vi "trial 1.vi"() -> ()   [LabVIEW 2013]
uses:
  <vilib>/vision/NI_Vision_Development_Module.lvlib
panel:
  in  "Contours 2":T1(array[cluster])
  in  "Global Rectangle 2":i32[](array[numeric])
  out "Contours":T1(array[cluster])
  out "Global Rectangle":i32[](array[numeric])
  out "Image 3":T2(plugin-control)
  in  "AVI File Path":path
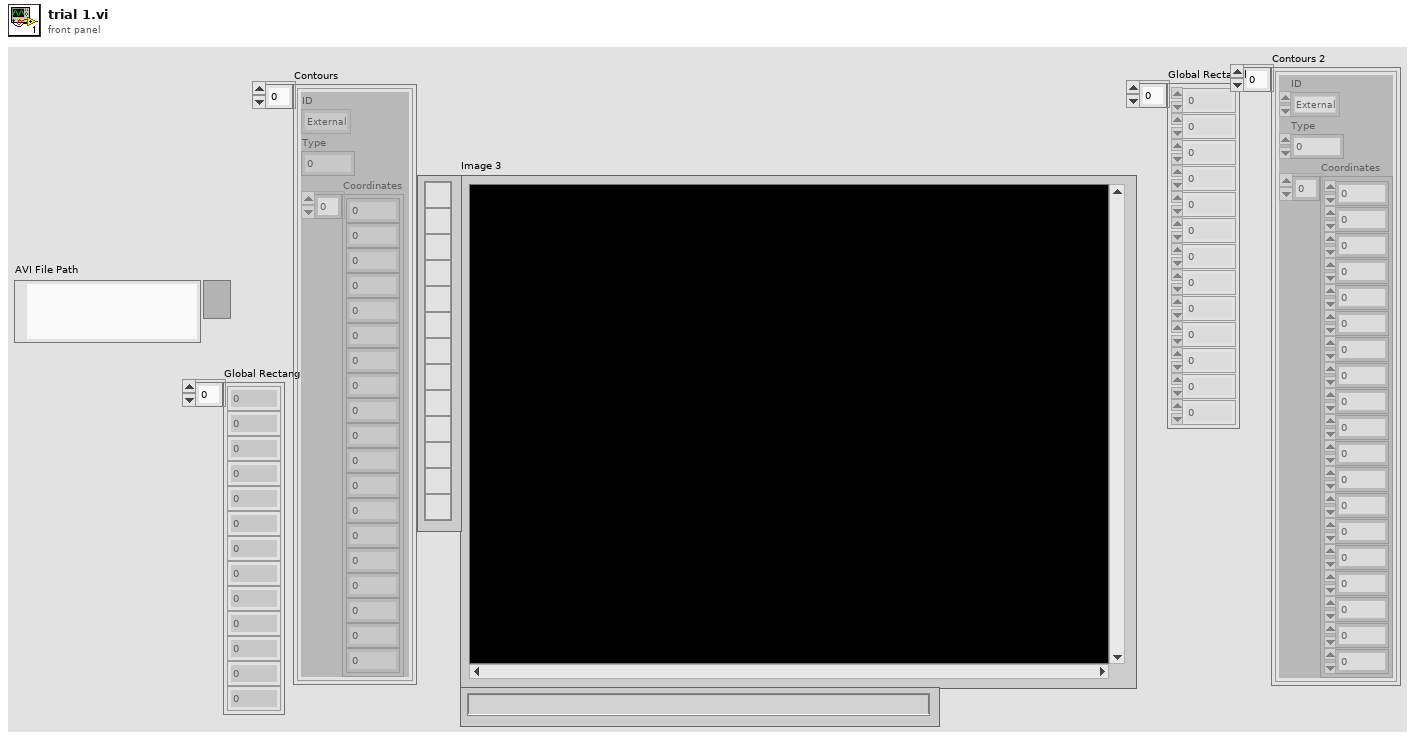
[diagram p1: front panel]
types:
  T1 = cluster{"ID":enum32{"External", "Internal"}, "Type":u32, "Coordinates":i32[]}[]
  T2 = typedef "IMAQ Image.ctl" = refnum<image>
  T3 = typedef "Image Type" = u32
  T4 = typedef "AviRefnum.ctl" = refnum<k1>
  T5 = typedef "ROI Descriptor" = cluster{"Global Rectangle":i32[], "Contours":cluster{"ID":enum32{"External", "Internal"}, "Type":u32, "Coordinates":i32[]}[]}
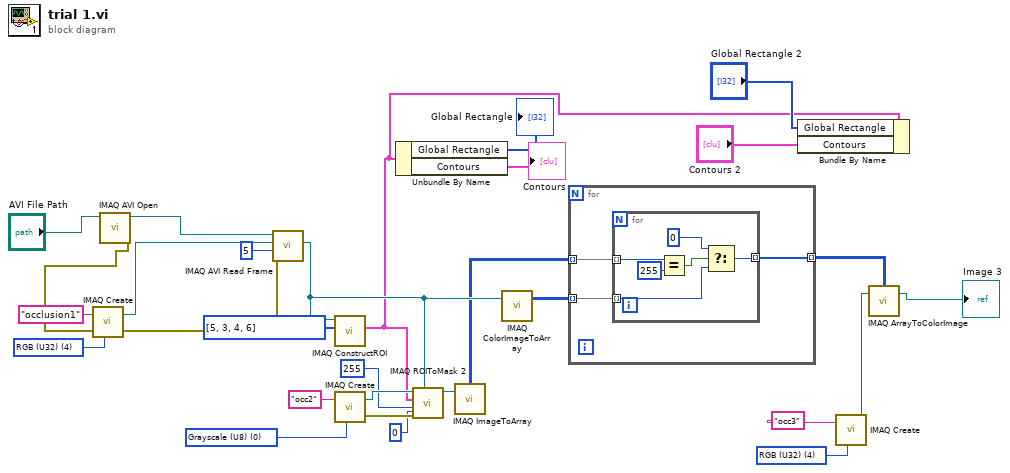
[diagram p0: block diagram]
diagram:
  w6 = u32[] [5, 3, 4, 6] items=["No Selection", "Point", "Line", "Rectangle", "Oval", "Polygon", "Freehand Region", "Annulus", "Zoom", "Pan", "Broken Line", "Freehand Line", "Rotated Rectangle"] ("Tools")
  w10 = T3 4 items=["Grayscale (U8)", "Grayscale (I16)", "Grayscale (SGL)", "Complex (CSG)", "RGB (U32)", "HSL (U32)", "RGB (U64)", "Grayscale (U16)"] ("Image Type")
  w20 = T3 0 items=["Grayscale (U8)", "Grayscale (I16)", "Grayscale (SGL)", "Complex (CSG)", "RGB (U32)", "HSL (U32)", "RGB (U64)", "Grayscale (U16)"] ("Image Type")
  w22 = T3 4 items=["Grayscale (U8)", "Grayscale (I16)", "Grayscale (SGL)", "Complex (CSG)", "RGB (U32)", "HSL (U32)", "RGB (U64)", "Grayscale (U16)"] ("Image Type")
  n1 = call "IMAQ AVI Open"("AVI Path"="AVI File Path") -> ("error out"=w27:errorcluster, "Avi Refnum"=w26:T4)  [unwired: 9 in]
  n2 = call "IMAQ Create"("Image Name"="occlusion1", "Image Type"=w22, "error in (no error)"=w27) -> ("New Image"=w24:T2, "error out"=w23:errorcluster)  [unwired: 2 in]
  n3 = call "IMAQ AVI Read Frame"("error in (no error)"=w23, "Frame Number"=u32 5, "Image"=w24, "Avi Refnum"=w26) -> ("Image Out"=w14:T2)  [unwired: 4 in, 3 out]
  n4 = call "IMAQ ConstructROI"("Tools"=w6, "Image"=w14) -> ("ROI Descriptor Out"=w1:T5)  [unwired: 6 in, 3 out]
  n5 = call "IMAQ Create"("Image Name"="occ2", "Image Type"=w20) -> ("New Image"=w18:T2, "error out"=w19:errorcluster)  [unwired: 3 in]
  n6 = Unbundle By Name(w1) -> ("Global Rectangle"=→"Global Rectangle":i32[], "Contours"=→"Contours":T1)
  n7 = call "IMAQ ROIToMask 2"("Background Value (0)"=0, "Image Model"=w14, "error in (no error)"=w19, "Filling Value (255)"=255, "ROI Descriptor"=w1, "Image"=w18) -> ("Image Out"=w15:T2)  [unwired: 3 in, 2 out]
  n8 = call "IMAQ ImageToArray"("Image"=w15) -> ("Image Pixels (U8)"=w13:u8[][])  [unwired: 3 in, 4 out]
  n9 = call "IMAQ ColorImageToArray"("Image"=w14) -> ("Image Pixels (U32)"=w12:u32[][])  [unwired: 3 in, 2 out]
  n10 = for {
    tunnel: w13 -> [w32] mode=indexing
    tunnel: w12 -> [w31] mode=indexing
    tunnel: [w30] -> w11 mode=indexing
    n11 = for {
      tunnel: w32 -> [w38] mode=indexing
      tunnel: w31 -> [w35] mode=indexing
      tunnel: [w33] -> w30 mode=indexing
      n12 = Equal?(x=w38, y=u8 255) -> (x = y?=w34:bool)
      n13 = Select(t=u32 0, s=w34, f=w35) -> (s? t:f=w33:u32)
    }
  }
  n14 = Bundle By Name(cluster=w1, "Global Rectangle"="Global Rectangle 2", "Contours"="Contours 2") -> ()  [unwired: 1 out]
  n15 = call "IMAQ Create"("Image Name"="occ3", "Image Type"=w10) -> ("New Image"=w8:T2)  [unwired: 3 in, 1 out]
  n16 = call "IMAQ ArrayToColorImage"("Image Pixels (U32)"=w11, "Image"=w8) -> ("Image Out"=→"Image 3":T2)  [unwired: 3 in, 1 out]
